vi "Copy Array to Image (Pixels).vi"(8 "error in (no error)":errorcluster, 10 "ARGB Image Destination":T1, 11 "(A)RGB Pixels Data":u8[][][](array[numeric])) -> (0 "error out":errorcluster, 3 "ARGB Image Destination (Duplicate)":T1)   [LabVIEW 2020, in "g_ar_toolkit.image.lvlib"]
uses:
  g_ar_toolkit.image.lvlib
  ARGB Image.ctl
  g_ar_toolkit.common/g_ar_toolkit.common.lvlib
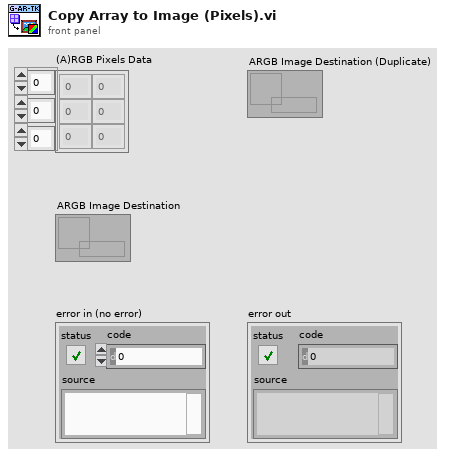
[diagram p1: front panel]
types:
  T1 = typedef "g_ar_toolkit.image.lvlib/ARGB Image.ctl" = refnum<data-value>
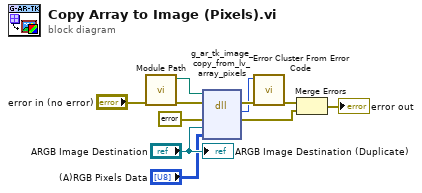
[diagram p0: block diagram]
diagram:
  n1 = call "Module Path.vi"("error in (no error)"="error in (no error)") -> ("error out"=w2:errorcluster, "Path"=w1:path)  [unwired: 9 in]
  n2 = dll-call lib="?" fn="g_ar_tk_image_copy_from_lv_array_pixels" ("g_ar_toolkit.*.*:g_ar_tk_image_copy_from_raw_memory")(path in=w1, error in=w2, "error_cluster"=errorcluster {"status"=FALSE, "code"=0, "source"=""} ("error constant"), "edvr_dst"="ARGB Image Destination", "array"="(A)RGB Pixels Data") -> (error out=w5:errorcluster, "MgErr"=w4:i32, "error_cluster"=w10:errorcluster)  [unwired: 3 in, 1 out]
  n3 = call <vilib>:"Error Cluster From Error Code.vi"("error in (no error)"=w5, "error code (0)"=w4) -> ("error out"=w6:errorcluster)  [unwired: 7 in]
  n4 = Merge Errors(w6, w10) -> (→"error out":errorcluster)
  "ARGB Image Destination (Duplicate)" <- "ARGB Image Destination"
